vi "Save Streamed Data.vi"(4 "Samples per Record":i32=51200, 5 "# Records to Skip (0)":i32, 6 "error in (no error)":errorcluster, 7 "Signals":dbl[][](array[numeric]), 8 "Destination File":path=path "C:/ScopeBinaryData.bin", 9 "# Records (-1)":i32=-1) -> (0 "error out":errorcluster, 3 "# Records Written":i32)   [LabVIEW 2013]
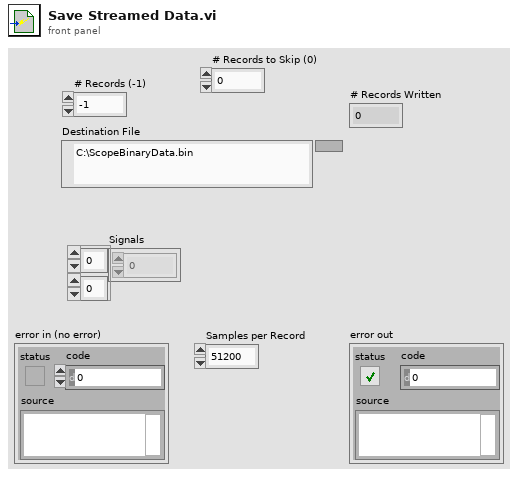
[diagram p1: front panel]
types:
  T1 = enum32{"CREATE_NEW (create)", "CREATE_ALWAYS (replace or create)", "OPEN_EXISTING (open)", "OPEN_ALWAYS (open or create)", "TRUNCATE_EXISTING (replace)"}
  T2 = enum16{"big-endian, network order", "native, host order", "little-endian"}
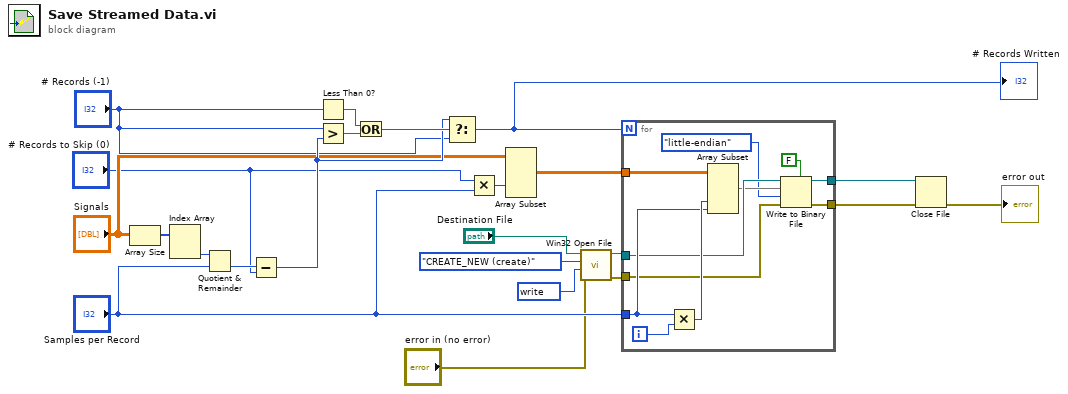
[diagram p0: block diagram]
diagram:
  w22 = u32 1073741824 items=["read"=2147483648, "write"=1073741824, "read & write"=3221225472, "execute"=536870912, "all"=268435456] ("desired access (read & write)")
  n1 = Array Size(array="Signals") -> (size(s)=w20:i32[])
  n2 = Index Array(array=w20) -> (element #2=w19:i32)  [unwired: 2 in, 1 out]
  n3 = Quotient & Remainder(x=w19, y="Samples per Record") -> (floor(x/y)=w18:i32)  [unwired: 1 out]
  n4 = Subtract(x=w18, y="# Records to Skip (0)") -> (x-y=w14:i32)
  n5 = Less Than 0?(x="# Records (-1)") -> (x < 0?=w17:bool)
  n6 = Greater?(x="# Records (-1)", y=w14) -> (0:w16:bool)
  n7 = Or(x=w17, y=w16) -> (x .or. y?=w15:bool)
  n8 = Select(t=w14, s=w15, f="# Records (-1)") -> (s? t:f=w12:i32)
  "# Records Written" <- w12
  n9 = Multiply(x="# Records to Skip (0)", y="Samples per Record") -> (x*y=w7:i32)
  n10 = Array Subset(array="Signals", index (col)=w7) -> (w10:dbl[][])  [unwired: 3 in]
  n11 = call "Win32 Open File.vi"("error in (no error)"="error in (no error)", "desired access (read & write)"=w22, "creation mode (open)"=T1."CREATE_NEW (create)", "file path"="Destination File") -> ("error out"=w5:errorcluster, "LabVIEW file refnum out"=w6:refnum<file>)  [unwired: 5 in, 1 out]
  n12 = for {
    N: w12 -> [_]
    tunnel: w10 -> [w33]
    tunnel: "Samples per Record" -> [w31]
    tunnel: w6 -> [w29]
    tunnel: w5 -> [w27]
    tunnel: [w26] -> w4
    tunnel: [w25] -> w2
    i -> [w34]
    n13 = Multiply(x=w31, y=w34) -> (x*y=w32:i32)
    n14 = Array Subset(array=w33, index (col)=w32, length (col)=w31) -> (w28:dbl[][])  [unwired: 2 in]
    n15 = Write to Binary File(file (use dialog)=w29, data=w28, error in=w27, 5:FALSE ("prepend array or string size? (T)"), 9:T2."little-endian" ("byte order (0:big-endian, network order)")) -> (refnum out=w26:refnum<file>, error out=w25:errorcluster)  [unwired: 1 in, 1 out]
  }
  n16 = Close File(refnum=w4, error in=w2) -> (error out=→"error out":errorcluster)  [unwired: 1 out]
